vi "getDescription.vi"(8 "error in (no error)":errorcluster, 11 "Camera in":refnum<class "Camera.lvclass">) -> (0 "error out":errorcluster, 2 "description":T1={"serial"=4294967295, "type"=0, "sub_type"=0, "interface_type"=65535, "bit_resolution"=0, "min_exposure_time_s"=nan, "max_exposure_time_s"=nan, "min_exposure_step_s"=nan, "min_delay_time_s"=nan, "max_delay_time_s"=nan, "min_delay_step_s"=nan, "min_width"=18446744073709551615, "min_height"=18446744073709551615, "max_width"=18446744073709551615, "max_height"=18446744073709551615, "roi_step_horz"=18446744073709551615, "roi_step_vert"=18446744073709551615, "roi_symmetric_horz"=FALSE, "roi_symmetric_vert"=FALSE, "has_timestamp_mode"=FALSE, "has_timestamp_mode_ascii_only"=FALSE, "pixelrate_vec"=[], "conversion_factor_vec"=[], "has_trigger_mode_extexpctrl"=FALSE, "has_acquire_mode"=FALSE, "has_ext_acquire_mode"=FALSE, "has_metadata_mode"=FALSE, "has_ram"=FALSE, "binning_horz_vec"=[], "binning_vert_vec"=[], "has_average_binning"=FALSE, "pixel_format_vec"=[]} {"conversion_factor_vec" format="%.2g"; "interface_type" items=["FireWire"=1, "GenICam"=3, "GigE"=5, "USB"=6, "CameraLinkME4"=7, "USB3"=8, "CLHS"=11, "All"=65535]}, 3 "Camera out":refnum<class "Camera.lvclass">)   [LabVIEW 2019, in "Camera.lvclass"]
doc: "Gets the camera description from the camera."
uses:
  Camera.lvclass
  Camera.lvclass/Camera.ctl
  pco.sdk/CameraDescription/CameraDescription.lvlib
  pco.sdk/ImageSensor/ImageSensor.lvlib
  pco.sdk/GeneralCameraControl/GeneralCameraControl.lvlib
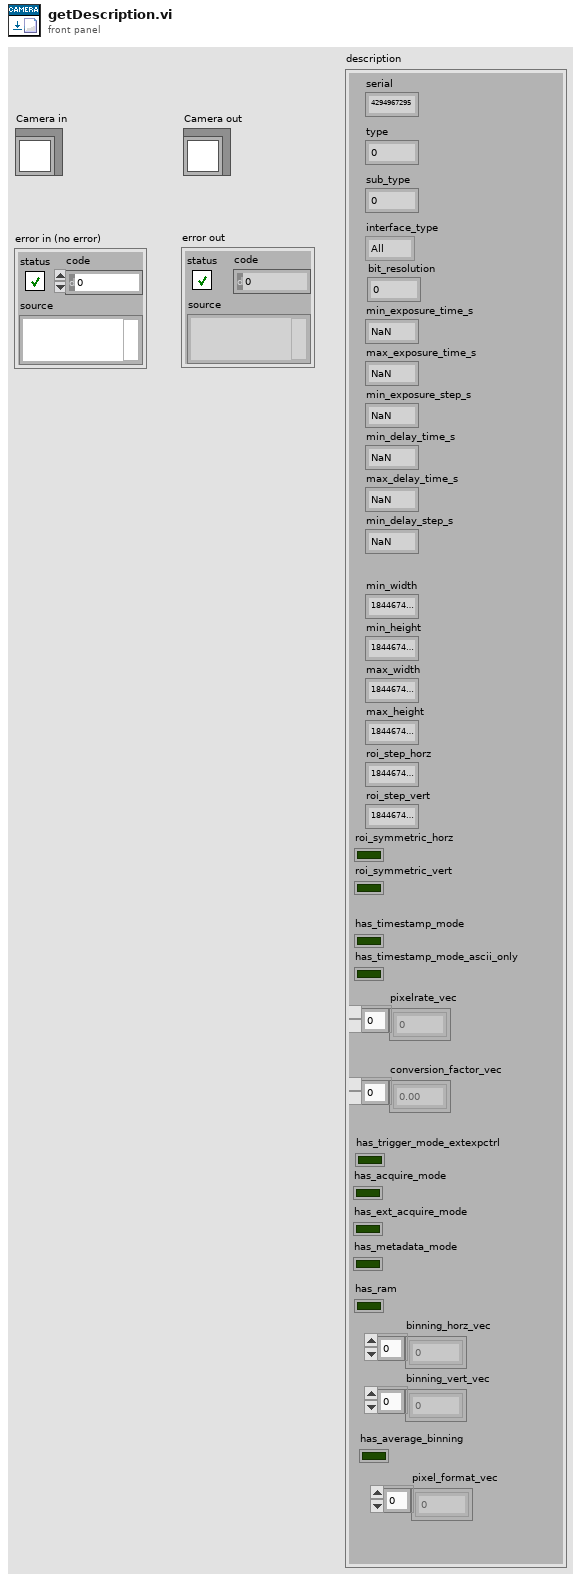
[diagram p1: front panel]
types:
  T1 = cluster{"serial":u32, "type":u16, "sub_type":u16, "interface_type":u16, "bit_resolution":u16, "min_exposure_time_s":dbl, "max_exposure_time_s":dbl, "min_exposure_step_s":dbl, "min_delay_time_s":dbl, "max_delay_time_s":dbl, "min_delay_step_s":dbl, "min_width":u64, "min_height":u64, "max_width":u64, "max_height":u64, "roi_step_horz":u64, "roi_step_vert":u64, "roi_symmetric_horz":bool, "roi_symmetric_vert":bool, "has_timestamp_mode":bool, "has_timestamp_mode_ascii_only":bool, "pixelrate_vec":u32[], "conversion_factor_vec":sgl[], "has_trigger_mode_extexpctrl":bool, "has_acquire_mode":bool, "has_ext_acquire_mode":bool, "has_metadata_mode":bool, "has_ram":bool, "binning_horz_vec":u16[], "binning_vert_vec":u16[], "has_average_binning":bool, "pixel_format_vec":u32[]}
  T2 = cluster{"serial":u32, "type":u16, "sub_type":u16, "interface_type":u16, "bit_resolution":u16, "min_exposure_time_s":dbl, "max_exposure_time_s":dbl, "min_exposure_step_s":dbl, "min_delay_time_s":dbl, "max_delay_time_s":dbl, "min_delay_step_s":dbl, "min_width":u64, "min_height":u64, "max_width":u64, "max_height":u64, "roi_step_horz":u64, "roi_step_vert":u64, "roi_symmetric_horz":bool, "roi_symmetric_vert":bool, "has_timestamp_mode":bool, "has_timestamp_mode_ascii_only":bool, "pixelrate_vec":u32[], "conversion_factor_vec":u32[], "has_trigger_mode_extexpctrl":bool, "has_acquire_mode":bool, "has_ext_acquire_mode":bool, "has_metadata_mode":bool, "has_ram":bool, "binning_horz_vec":u16[], "binning_vert_vec":u16[], "has_average_binning":bool, "pixel_format_vec":u32[]}
  T3 = enum16{"SETUP_TYPE_SHUTTERMODE", "SETUP_TYPE_PIXELFORMAT", "SETUP_TYPE_SENSOR_DYNRES"}
  T4 = cluster{"wSensorTypeDESC":u16, "wSensorSubTypeDESC":u16, "wMaxHorzResStdDESC":u16, "wMaxVertResStdDESC":u16, "wMaxHorzResExtDESC":u16, "wMaxVertResExtDESC":u16, "wDynResDESC":u16, "wMaxBinHorzDESC":u16, "wBinHorzSteppingDESC":u16, "wMaxBinVertDESC":u16, "wBinVertSteppingDESC":u16, "wRoiHorStepsDESC":u16, "wRoiVertStepsDESC":u16, "wNumADCsDESC":u16, "wMinSizeHorzDESC":u16, "dwPixelRateDESC":u32[], "wConvFactDESC":u16[], "sCoolingSetpoints":i16[], "wSoftRoiHorStepsDESC":u16, "wSoftRoiVertStepsDESC":u16, "wIRDESC":u16, "wMinSizeVertDESC":u16, "dwMinDelayDESC":u32, "dwMaxDelayDESC":u32, "dwMinDelayStepDESC":u32, "dwMinExposureDESC":u32, "dwMaxExposureDESC":u32, "dwMinExposureStepDESC":u32, "dwMinDelayIRDESC":u32, "dwMaxDelayIRDESC":u32, "dwMinExposureIRDESC":u32, "dwMaxExposureIRDESC":u32, "wTimeTableDESC":u16, "wDoubleImageDESC":u16, "sMinCoolSetDESC":i16, "sMaxCoolSetDESC":i16, "sDefaultCoolSetDESC":i16, "wPowerDownModeDESC":u16, "wOffsetRegulationDESC":u16, "wColorPatternDESC":u16, "wPatternTypeDESC":u16, "wNumCoolingSetpoints":u16, "dwGeneralCapsDESC1":u32, "dwGeneralCapsDESC2":u32, "dwExtSyncFrequency":u32[], "dwGeneralCapsDESC3":u32, "dwGeneralCapsDESC4":u32}
  T5 = cluster{"wDarkOffsetDESC3":u16, "dwGeneralCapsDESC3_1":u32, "dwGeneralCapsDESC3_2":u32, "dwGeneralCapsDESC3_3":u32, "dwGeneralCapsDESC3_4":u32, "wMinHorzResStdDESC3":u16, "wMinVertResStdDESC3":u16, "wMinHorzResExtDESC3":u16, "wMinVertResExtDESC3":u16, "dPixelsize_horzDESC3_um":dbl, "dPixelsize_vertDESC3_um":dbl, "dMinSensorTempWarningDESC3_C":dbl, "dMaxSensorTempWarningDESC3_C":dbl, "dMinCameraTempWarningDESC3_C":dbl, "dMaxCameraTempWarningDESC3_C":dbl, "dMinPowerTempWarningDESC3_C":dbl, "dMaxPowerTempWarningDESC3_C":dbl, "dMinPowerVoltageWarningDESC3_V":dbl, "dMaxPowerVoltageWarningDESC3_V":dbl, "dMinSensorTempErrorDESC3_C":dbl, "dMaxSensorTempErrorDESC3_C":dbl, "dMinCameraTempErrorDESC3_C":dbl, "dMaxCameraTempErrorDESC3_C":dbl, "dMinPowerTempErrorDESC3_C":dbl, "dMaxPowerTempErrorDESC3_C":dbl, "dMinPowerVoltageErrorDESC3_V":dbl, "dMaxPowerVoltageErrorDESC3_V":dbl}
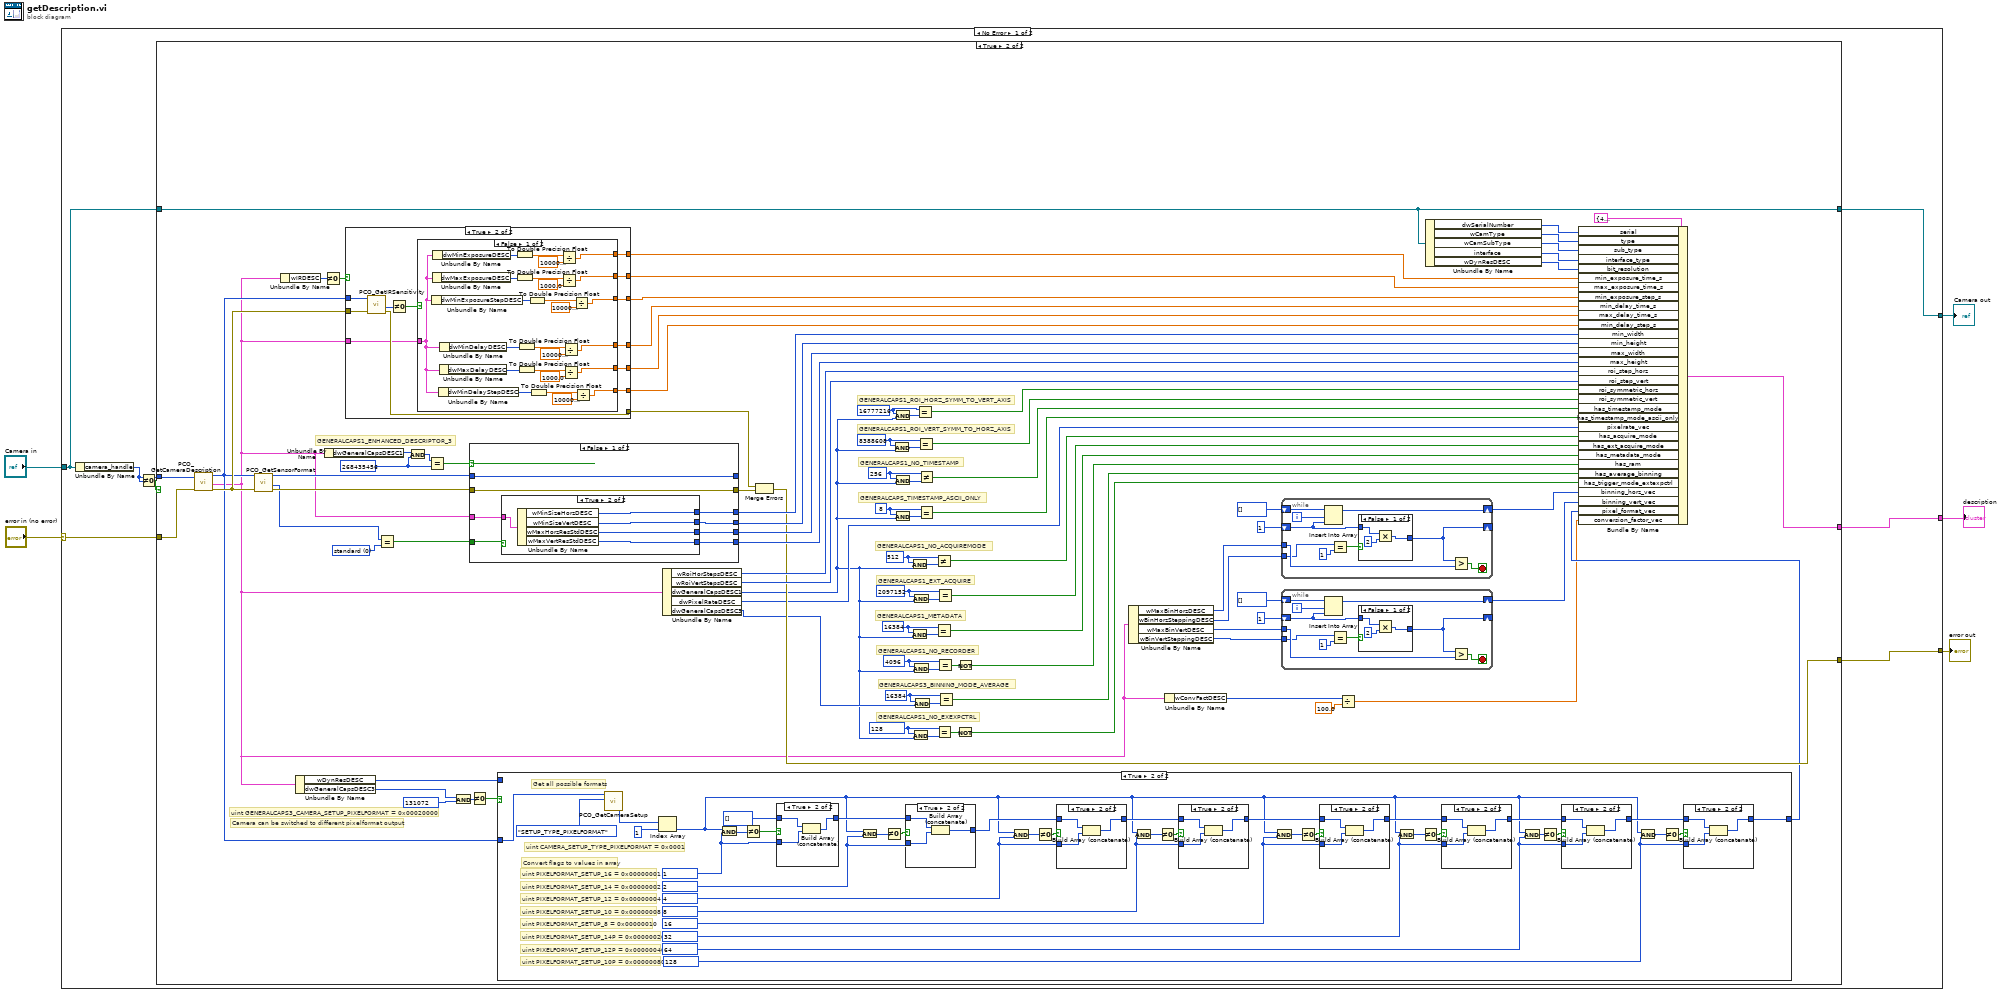
[diagram p0: block diagram]
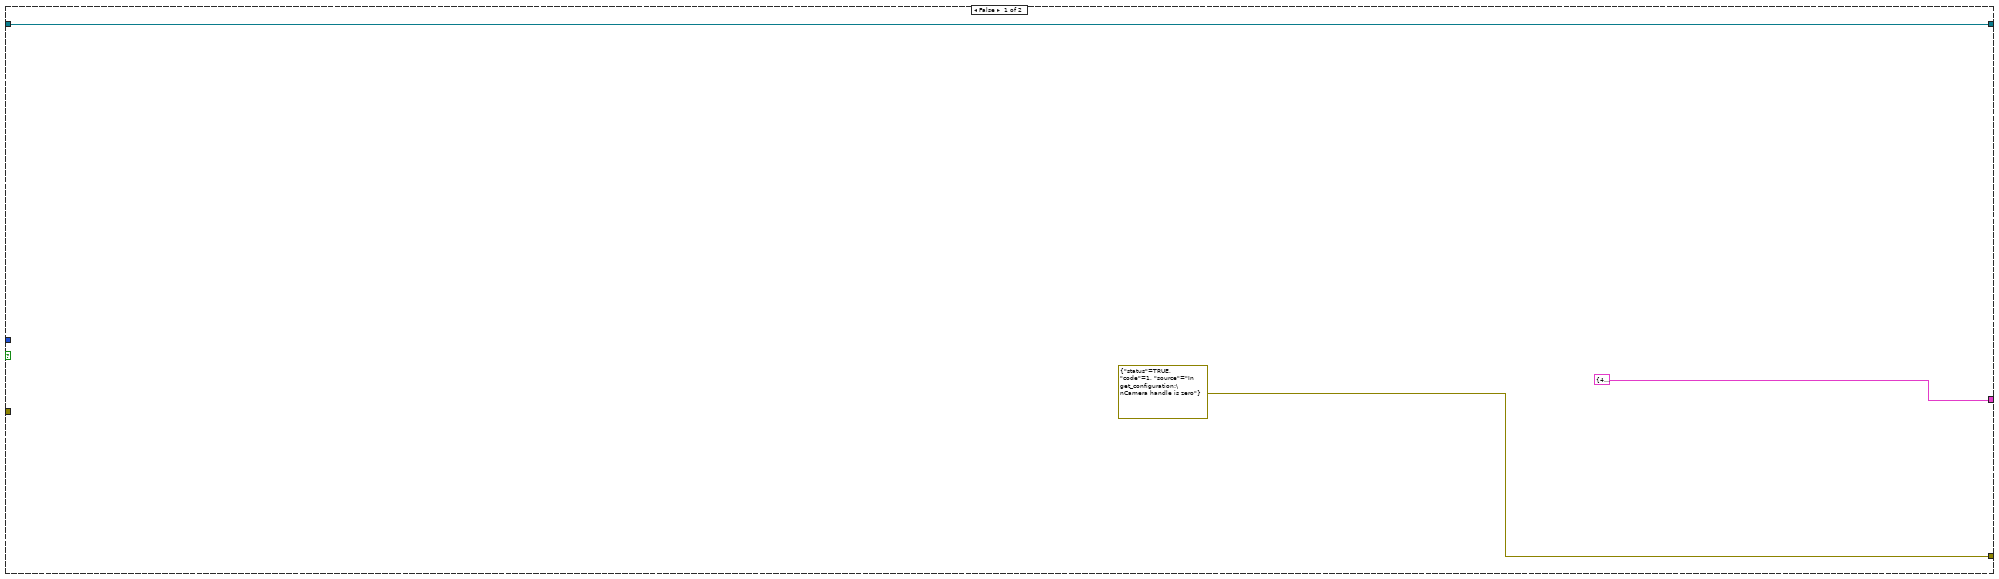
[diagram p2: hidden frame]
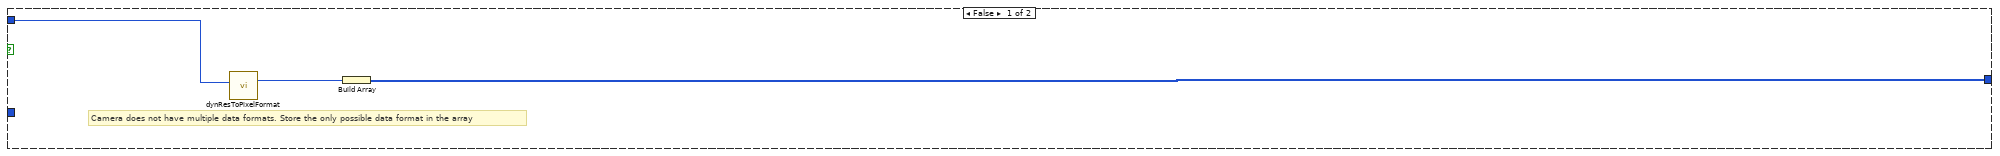
[diagram p3: hidden frame]
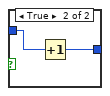
[diagram p12: hidden frame]
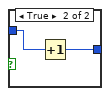
[diagram p13: hidden frame]
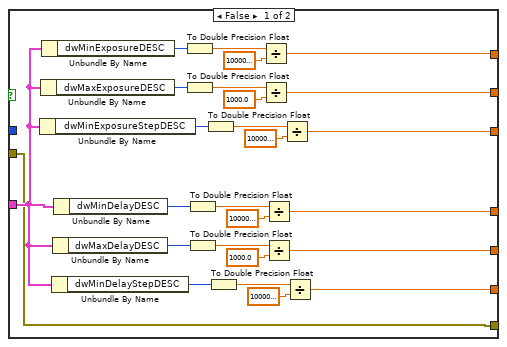
[diagram p14: hidden frame]
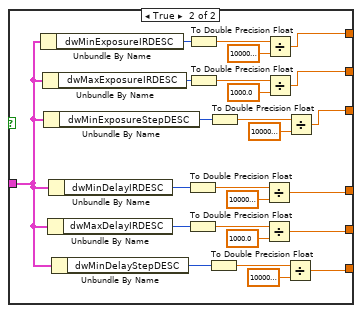
[diagram p15: hidden frame]
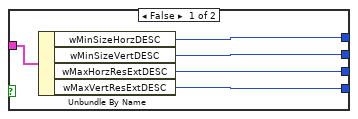
[diagram p16: hidden frame]
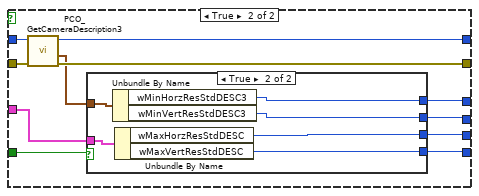
[diagram p17: hidden frame]
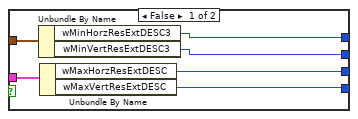
[diagram p18: hidden frame]
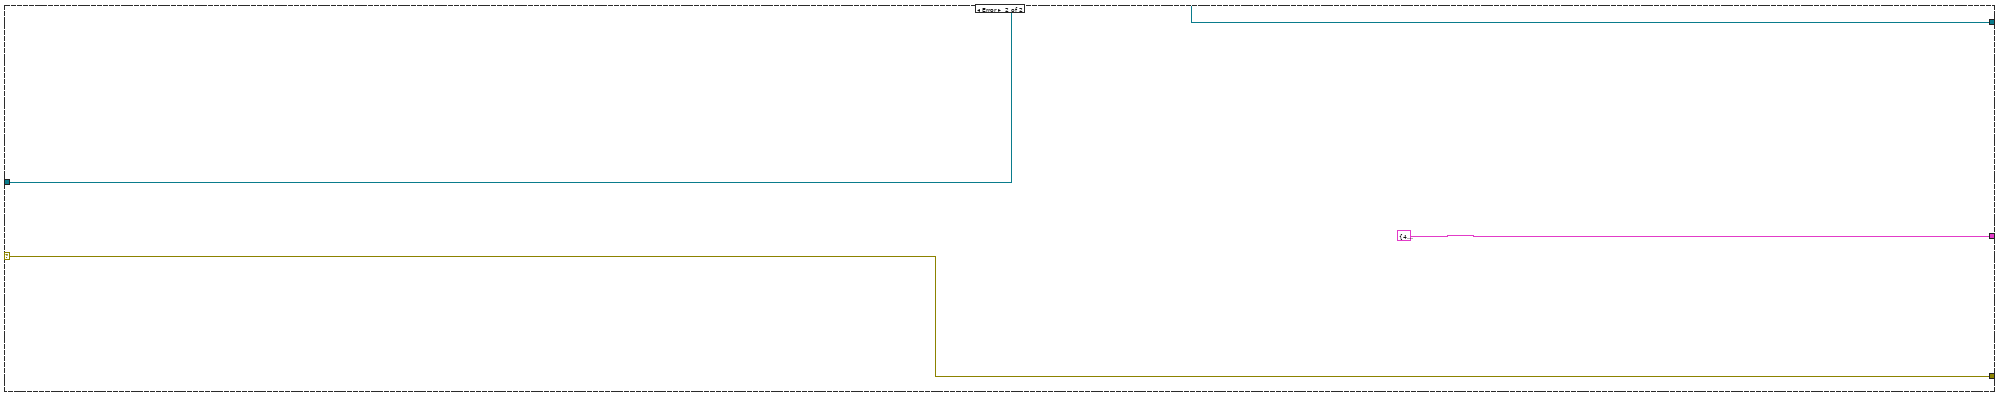
[diagram p19: hidden frame]
diagram:
  n1 = case shown="No Error" "error in (no error)" {
    selector: "error in (no error)" -> [w9 w343]
    tunnel: [w11 w343] -> w4
    tunnel: [w6 w342] -> w2
    tunnel: "Camera in" -> [w8 w342]
    tunnel: [w7 T2 {"serial"=4294967295, "type"=0, "sub_type"=0, "interface_type"=65535, "bit_resolution"=0, "min_exposure_time_s"=nan, "max_exposure_time_s"=nan, "min_exposure_step_s"=nan, "min_delay_time_s"=nan, "max_delay_time_s"=nan, "min_delay_step_s"=nan, "min_width"=18446744073709551615, "min_height"=18446744073709551615, "max_width"=18446744073709551615, "max_height"=18446744073709551615, "roi_step_horz"=18446744073709551615, "roi_step_vert"=18446744073709551615, "roi_symmetric_horz"=FALSE, "roi_symmetric_vert"=FALSE, "has_timestamp_mode"=FALSE, "has_timestamp_mode_ascii_only"=FALSE, "pixelrate_vec"=[], "conversion_factor_vec"=[], "has_trigger_mode_extexpctrl"=FALSE, "has_acquire_mode"=FALSE, "has_ext_acquire_mode"=FALSE, "has_metadata_mode"=FALSE, "has_ram"=FALSE, "binning_horz_vec"=[], "binning_vert_vec"=[], "has_average_binning"=FALSE, "pixel_format_vec"=[]} ("description")] -> w1
    frame No Error {
      n2 = Unbundle By Name(w8) -> ("camera_handle"=w10:u64)
      n3 = Not Equal To 0?(x=w10) -> (x != 0?=w12:bool)
      n4 = case shown="True" w12 {
        tunnel: [errorcluster {"status"=TRUE, "code"=1, "source"="In get_configuration:\nCamera handle is zero"} ("error constant") w68] -> w11
        tunnel: w10 -> [_ w108]
        tunnel: w9 -> [_ w107]
        tunnel: w8 -> [w14 w49]
        tunnel: [T2 {"serial"=4294967295, "type"=0, "sub_type"=0, "interface_type"=65535, "bit_resolution"=0, "min_exposure_time_s"=nan, "max_exposure_time_s"=nan, "min_exposure_step_s"=nan, "min_delay_time_s"=nan, "max_delay_time_s"=nan, "min_delay_step_s"=nan, "min_width"=18446744073709551615, "min_height"=18446744073709551615, "max_width"=18446744073709551615, "max_height"=18446744073709551615, "roi_step_horz"=18446744073709551615, "roi_step_vert"=18446744073709551615, "roi_symmetric_horz"=FALSE, "roi_symmetric_vert"=FALSE, "has_timestamp_mode"=FALSE, "has_timestamp_mode_ascii_only"=FALSE, "pixelrate_vec"=[], "conversion_factor_vec"=[], "has_trigger_mode_extexpctrl"=FALSE, "has_acquire_mode"=FALSE, "has_ext_acquire_mode"=FALSE, "has_metadata_mode"=FALSE, "has_ram"=FALSE, "binning_horz_vec"=[], "binning_vert_vec"=[], "has_average_binning"=FALSE, "pixel_format_vec"=[]} ("description") w35] -> w7
        tunnel: [w14 w49] -> w6
        frame False {
        }
        frame True {
          w24 = u32 128 ("dwGeneralCapsDESC1")
          w39 = u32 16384 ("dwGeneralCapsDESC1")
          w42 = u32 4096 ("dwGeneralCapsDESC1")
          w60 = u32 16384 ("dwGeneralCapsDESC1")
          w62 = u32 2097152 ("dwGeneralCapsDESC1")
          w66 = u32 512 ("dwGeneralCapsDESC1")
          w72 = u32 8 ("dwGeneralCapsDESC1")
          w76 = u32 256 ("dwGeneralCapsDESC1")
          w81 = u32 8388608 ("dwGeneralCapsDESC1")
          w80 = u32 16777216 ("dwGeneralCapsDESC1")
          w100 = u16 0 items=["standard", "extended"] ("wSensor")
          w104 = u32 268435456 ("dwGeneralCapsDESC1")
          # "GENERALCAPS1_NO_EXEXPCTRL"
          # "Camera can be switched to different pixelformat output"
          # "uint GENERALCAPS3_CAMERA_SETUP_PIXELFORMAT = 0x00020000"
          # "GENERALCAPS3_BINNING_MODE_AVERAGE"
          # "GENERALCAPS1_NO_RECORDER"
          # "GENERALCAPS1_METADATA"
          # "GENERALCAPS1_EXT_ACQUIRE"
          # "GENERALCAPS1_NO_ACQUIREMODE"
          # "GENERALCAPS_TIMESTAMP_ASCII_ONLY"
          # "GENERALCAPS1_NO_TIMESTAMP"
          # "GENERALCAPS1_ROI_VERT_SYMM_TO_HORZ_AXIS"
          # "GENERALCAPS1_ROI_HORZ_SYMM_TO_VERT_AXIS"
          # "GENERALCAPS1_ENHANCED_DESCRIPTOR_3"
          n5 = call "PCO_GetCameraDescription.vi"("error in (no error)"=w107, "ph"=w108) -> ("error out"=w90:errorcluster, "strDescription"=w19:T4, "ph out"=w30:u64)  [unwired: 6 in, 1 out]
          n6 = call "PCO_GetSensorFormat.vi"("error in (no error)"=w90, "ph"=w30) -> ("error out"=w102:errorcluster, "wSensor"=w99:u16, "ph out"=w101:u64)  [unwired: 6 in, 1 out]
          n7 = Unbundle By Name(w19) -> ("wIRDESC"=w98:u16)
          n8 = Unbundle By Name(w19) -> ("wDynResDESC"=w29:u16, "dwGeneralCapsDESC3"=w34:u32)
          n9 = Not Equal To 0?(x=w98) -> (x != 0?=w97:bool)
          n10 = Unbundle By Name(w19) -> ("dwGeneralCapsDESC1"=w106:u32)
          n11 = case shown="True" w97 {
            tunnel: w30 -> [_ w249]
            tunnel: w90 -> [w212 w248]
            tunnel: w19 -> [w218 w238]
            tunnel: [w234 w244] -> w96
            tunnel: [w217 w243] -> w95
            tunnel: [w216 w242] -> w94
            tunnel: [w215 w241] -> w93
            tunnel: [w214 w240] -> w92
            tunnel: [w213 w239] -> w91
            tunnel: [w212 w246] -> w70
            frame False {
              n12 = Unbundle By Name(w218) -> ("dwMinExposureStepDESC"=w228:u32)
              n13 = Unbundle By Name(w218) -> ("dwMaxExposureDESC"=w231:u32)
              n14 = Unbundle By Name(w218) -> ("dwMinExposureDESC"=w237:u32)
              n15 = Unbundle By Name(w218) -> ("dwMinDelayStepDESC"=w219:u32)
              n16 = Unbundle By Name(w218) -> ("dwMaxDelayDESC"=w222:u32)
              n17 = Unbundle By Name(w218) -> ("dwMinDelayDESC"=w227:u32)
              n18 = To Double Precision Float(number=w237) -> (double precision float=w236:dbl)
              n19 = To Double Precision Float(number=w231) -> (double precision float=w233:dbl)
              n20 = To Double Precision Float(number=w227) -> (double precision float=w226:dbl)
              n21 = To Double Precision Float(number=w222) -> (double precision float=w224:dbl)
              n22 = To Double Precision Float(number=w228) -> (double precision float=w230:dbl)
              n23 = To Double Precision Float(number=w219) -> (double precision float=w221:dbl)
              n24 = Divide(x=w236, y=1000000000.0) -> (x/y=w234:dbl)
              n25 = Divide(x=w233, y=1000.0) -> (x/y=w217:dbl)
              n26 = Divide(x=w226, y=1000000000.0) -> (x/y=w215:dbl)
              n27 = Divide(x=w224, y=1000.0) -> (x/y=w214:dbl)
              n28 = Divide(x=w230, y=1000000000.0) -> (x/y=w216:dbl)
              n29 = Divide(x=w221, y=1000000000.0) -> (x/y=w213:dbl)
            }
            frame True {
              n30 = call "PCO_GetIRSensitivity.vi"("error in (no error)"=w248, "ph"=w249) -> ("error out"=w246:errorcluster, "wIR"=w247:u16)  [unwired: 6 in, 2 out]
              n31 = Not Equal To 0?(x=w247) -> (x != 0?=w245:bool)
              n32 = case shown="False" w245 {
                tunnel: [w262 w286] -> w244
                tunnel: [w261 w285] -> w243
                tunnel: [w260 w284] -> w242
                tunnel: [w259 w283] -> w241
                tunnel: [w258 w282] -> w240
                tunnel: [w257 w281] -> w239
                tunnel: w238 -> [w250 w287]
                frame False {
                  n33 = Unbundle By Name(w250) -> ("dwMinExposureStepDESC"=w269:u32)
                  n34 = Unbundle By Name(w250) -> ("dwMaxExposureDESC"=w271:u32)
                  n35 = Unbundle By Name(w250) -> ("dwMinExposureDESC"=w274:u32)
                  n36 = Unbundle By Name(w250) -> ("dwMinDelayStepDESC"=w263:u32)
                  n37 = Unbundle By Name(w250) -> ("dwMaxDelayDESC"=w265:u32)
                  n38 = Unbundle By Name(w250) -> ("dwMinDelayDESC"=w268:u32)
                  n39 = To Double Precision Float(number=w274) -> (double precision float=w273:dbl)
                  n40 = To Double Precision Float(number=w271) -> (double precision float=w272:dbl)
                  n41 = To Double Precision Float(number=w268) -> (double precision float=w267:dbl)
                  n42 = To Double Precision Float(number=w265) -> (double precision float=w266:dbl)
                  n43 = To Double Precision Float(number=w269) -> (double precision float=w270:dbl)
                  n44 = To Double Precision Float(number=w263) -> (double precision float=w264:dbl)
                  n45 = Divide(x=w273, y=1000000000.0) -> (x/y=w262:dbl)
                  n46 = Divide(x=w272, y=1000.0) -> (x/y=w261:dbl)
                  n47 = Divide(x=w267, y=1000000000.0) -> (x/y=w259:dbl)
                  n48 = Divide(x=w266, y=1000.0) -> (x/y=w258:dbl)
                  n49 = Divide(x=w270, y=1000000000.0) -> (x/y=w260:dbl)
                  n50 = Divide(x=w264, y=1000000000.0) -> (x/y=w257:dbl)
                }
                frame True {
                  n51 = Unbundle By Name(w287) -> ("dwMinExposureIRDESC"=w299:u32)
                  n52 = Unbundle By Name(w287) -> ("dwMaxExposureIRDESC"=w296:u32)
                  n53 = Unbundle By Name(w287) -> ("dwMinExposureStepDESC"=w294:u32)
                  n54 = Unbundle By Name(w287) -> ("dwMaxDelayIRDESC"=w290:u32)
                  n55 = Unbundle By Name(w287) -> ("dwMinDelayIRDESC"=w293:u32)
                  n56 = Unbundle By Name(w287) -> ("dwMinDelayStepDESC"=w288:u32)
                  n57 = To Double Precision Float(number=w293) -> (double precision float=w292:dbl)
                  n58 = To Double Precision Float(number=w290) -> (double precision float=w291:dbl)
                  n59 = To Double Precision Float(number=w299) -> (double precision float=w298:dbl)
                  n60 = To Double Precision Float(number=w296) -> (double precision float=w297:dbl)
                  n61 = To Double Precision Float(number=w288) -> (double precision float=w289:dbl)
                  n62 = To Double Precision Float(number=w294) -> (double precision float=w295:dbl)
                  n63 = Divide(x=w292, y=1000000000.0) -> (x/y=w283:dbl)
                  n64 = Divide(x=w291, y=1000.0) -> (x/y=w282:dbl)
                  n65 = Divide(x=w298, y=1000000000.0) -> (x/y=w286:dbl)
                  n66 = Divide(x=w297, y=1000.0) -> (x/y=w285:dbl)
                  n67 = Divide(x=w289, y=1000000000.0) -> (x/y=w281:dbl)
                  n68 = Divide(x=w295, y=1000000000.0) -> (x/y=w284:dbl)
                }
              }
            }
          }
          n69 = Equal?(x=w99, y=w100) -> (x = y?=w89:bool)
          n70 = And(x=w106, y=w104) -> (x .and. y?=w105:u32)
          n71 = Equal?(x=w105, y=w104) -> (x = y?=w103:bool)
          n72 = And(x=w34, y=u32 131072) -> (x .and. y?=w32:u32)
          n73 = case shown="False" w103 {
            tunnel: w102 -> [w307 w328]
            tunnel: w101 -> [w306 w327]
            tunnel: w19 -> [w304 w323]
            tunnel: [w307 w325] -> w69
            tunnel: [w306 w326] -> _
            tunnel: w89 -> [w305 w324]
            tunnel: [w303 w321] -> w88
            tunnel: [w302 w320] -> w87
            tunnel: [w301 w319] -> w86
            tunnel: [w300 w318] -> w85
            frame False {
              n74 = case shown="True" w305 {
                tunnel: w304 -> [w312 w317]
                tunnel: [w308 w316] -> w303
                tunnel: [w309 w315] -> w302
                tunnel: [w310 w314] -> w301
                tunnel: [w311 w313] -> w300
                frame False {
                  n75 = Unbundle By Name(w312) -> ("wMinSizeHorzDESC"=w308:u16, "wMinSizeVertDESC"=w309:u16, "wMaxHorzResExtDESC"=w310:u16, "wMaxVertResExtDESC"=w311:u16)
                }
                frame True {
                  n76 = Unbundle By Name(w317) -> ("wMinSizeHorzDESC"=w316:u16, "wMinSizeVertDESC"=w315:u16, "wMaxHorzResStdDESC"=w314:u16, "wMaxVertResStdDESC"=w313:u16)
                }
              }
            }
            frame True {
              n77 = call "PCO_GetCameraDescription3.vi"("error in (no error)"=w328, "ph"=w327) -> ("error out"=w325:errorcluster, "strDescription"=w322:T5, "ph out"=w326:u64)  [unwired: 6 in, 1 out]
              n78 = case shown="True" w324 {
                tunnel: w323 -> [w333 w340]
                tunnel: [w329 w336] -> w321
                tunnel: [w330 w335] -> w320
                tunnel: [w331 w339] -> w319
                tunnel: [w332 w338] -> w318
                tunnel: w322 -> [w334 w337]
                frame False {
                  n79 = Unbundle By Name(w334) -> ("wMinHorzResExtDESC3"=w329:u16, "wMinVertResExtDESC3"=w330:u16)
                  n80 = Unbundle By Name(w333) -> ("wMaxHorzResExtDESC"=w331:u16, "wMaxVertResExtDESC"=w332:u16)
                }
                frame True {
                  n81 = Unbundle By Name(w337) -> ("wMinHorzResStdDESC3"=w336:u16, "wMinVertResStdDESC3"=w335:u16)
                  n82 = Unbundle By Name(w340) -> ("wMaxHorzResStdDESC"=w339:u16, "wMaxVertResStdDESC"=w338:u16)
                }
              }
            }
          }
          n83 = Not Equal To 0?(x=w32) -> (x != 0?=w31:bool)
          n84 = case shown="True" w31 {
            tunnel: w30 -> [_ w147]
            tunnel: [w109 w113] -> w28
            tunnel: w29 -> [w111 _]
            frame False {
              # "Camera does not have multiple data formats. Store the only possible data format in the array"
              n85 = call "dynResToPixelFormat.vi"("dyn_res"=w111) -> ("PixelFormat"=w110:u32)  [unwired: 9 in, 1 out]
              n86 = Build Array(w110) -> (w109:u32[])
            }
            frame True {
              w114 = u32 128
              w115 = u32 64
              w123 = u32 32
              w124 = u32 16
              w131 = u32 8
              w135 = u32 4
              w140 = u32 2
              w143 = u32 1
              # "Convert flags to values in array"
              # "Get all possible formats"
              # "uint PIXELFORMAT_SETUP_10P = 0x00000080"
              # "uint PIXELFORMAT_SETUP_12P = 0x00000040"
              # "uint PIXELFORMAT_SETUP_14P = 0x00000020"
              # "uint PIXELFORMAT_SETUP_8 = 0x00000010"
              # "uint PIXELFORMAT_SETUP_10 = 0x00000008"
              # "uint PIXELFORMAT_SETUP_12 = 0x00000004"
              # "uint PIXELFORMAT_SETUP_14 = 0x00000002"
              # "uint PIXELFORMAT_SETUP_16 = 0x00000001"
              # "uint CAMERA_SETUP_TYPE_PIXELFORMAT = 0x0001"
              n87 = call "PCO_GetCameraSetup.vi"("wTypeIn"=T3."SETUP_TYPE_PIXELFORMAT", "ph"=w147) -> ("dwSetup"=w149:u32[])  [unwired: 5 in, 4 out]
              n88 = Index Array(array=w149, index=1) -> (element=w116:u32)
              n89 = And(x=w116, y=w143) -> (x .and. y?=w146:u32)
              n90 = Not Equal To 0?(x=w146) -> (x != 0?=w145:bool)
              n91 = case shown="True" w145 {
                tunnel: u32[] [] -> [w178 w181]
                tunnel: w143 -> [_ w180]
                tunnel: [w178 w179] -> w139
                frame False {
                }
                frame True {
                  n92 = Build Array (concatenate)(w181, w180) -> (w179:u32[])
                }
              }
              n93 = And(x=w116, y=w140) -> (x .and. y?=w142:u32)
              n94 = Not Equal To 0?(x=w142) -> (x != 0?=w141:bool)
              n95 = case shown="True" w141 {
                tunnel: w139 -> [w174 w177]
                tunnel: w140 -> [_ w176]
                tunnel: [w174 w175] -> w136
                frame False {
                }
                frame True {
                  n96 = Build Array (concatenate)(w177, w176) -> (w175:u32[])
                }
              }
              n97 = And(x=w116, y=w135) -> (x .and. y?=w137:u32)
              n98 = Not Equal To 0?(x=w137) -> (x != 0?=w138:bool)
              n99 = case shown="True" w138 {
                tunnel: w136 -> [w170 w173]
                tunnel: w135 -> [_ w172]
                tunnel: [w170 w171] -> w132
                frame False {
                }
                frame True {
                  n100 = Build Array (concatenate)(w173, w172) -> (w171:u32[])
                }
              }
              n101 = And(x=w116, y=w131) -> (x .and. y?=w134:u32)
              n102 = Not Equal To 0?(x=w134) -> (x != 0?=w133:bool)
              n103 = case shown="True" w133 {
                tunnel: w132 -> [w166 w169]
                tunnel: w131 -> [_ w168]
                tunnel: [w166 w167] -> w125
                frame False {
                }
                frame True {
                  n104 = Build Array (concatenate)(w169, w168) -> (w167:u32[])
                }
              }
              n105 = And(x=w116, y=w124) -> (x .and. y?=w127:u32)
              n106 = Not Equal To 0?(x=w127) -> (x != 0?=w126:bool)
              n107 = case shown="True" w126 {
                tunnel: w125 -> [w162 w165]
                tunnel: w124 -> [_ w164]
                tunnel: [w162 w163] -> w130
                frame False {
                }
                frame True {
                  n108 = Build Array (concatenate)(w165, w164) -> (w163:u32[])
                }
              }
              n109 = And(x=w116, y=w123) -> (x .and. y?=w128:u32)
              n110 = Not Equal To 0?(x=w128) -> (x != 0?=w129:bool)
              n111 = case shown="True" w129 {
                tunnel: w130 -> [w158 w161]
                tunnel: w123 -> [_ w160]
                tunnel: [w158 w159] -> w117
                frame False {
                }
                frame True {
                  n112 = Build Array (concatenate)(w161, w160) -> (w159:u32[])
                }
              }
              n113 = And(x=w116, y=w115) -> (x .and. y?=w121:u32)
              n114 = Not Equal To 0?(x=w121) -> (x != 0?=w122:bool)
              n115 = case shown="True" w122 {
                tunnel: w117 -> [w154 w157]
                tunnel: w115 -> [_ w156]
                tunnel: [w154 w155] -> w118
                frame False {
                }
                frame True {
                  n116 = Build Array (concatenate)(w157, w156) -> (w155:u32[])
                }
              }
              n117 = And(x=w116, y=w114) -> (x .and. y?=w120:u32)
              n118 = Not Equal To 0?(x=w120) -> (x != 0?=w119:bool)
              n119 = case shown="True" w119 {
                tunnel: w118 -> [w150 w153]
                tunnel: w114 -> [_ w152]
                tunnel: [w150 w151] -> w113
                frame False {
                }
                frame True {
                  n120 = Build Array (concatenate)(w153, w152) -> (w151:u32[])
                }
              }
            }
          }
          n121 = Unbundle By Name(w19) -> ("wRoiHorStepsDESC"=w84:u16, "wRoiVertStepsDESC"=w83:u16, "dwGeneralCapsDESC1"=w22:u32, "dwPixelRateDESC"=w67:u32[], "dwGeneralCapsDESC3"=w37:u32)
          n122 = Merge Errors(w70, w69) -> (w68:errorcluster)
          n123 = And(x=w81, y=w22) -> (x .and. y?=w82:u32)
          n124 = And(x=w80, y=w22) -> (x .and. y?=w79:u32)
          n125 = And(x=w76, y=w22) -> (x .and. y?=w75:u32)
          n126 = And(x=w72, y=w22) -> (x .and. y?=w73:u32)
          n127 = And(x=w66, y=w22) -> (x .and. y?=w65:u32)
          n128 = And(x=w60, y=w22) -> (x .and. y?=w59:u32)
          n129 = And(x=w24, y=w22) -> (x .and. y?=w23:u32)
          n130 = And(x=w62, y=w22) -> (x .and. y?=w63:u32)
          n131 = And(x=w42, y=w22) -> (x .and. y?=w43:u32)
          n132 = And(x=w39, y=w37) -> (x .and. y?=w38:u32)
          n133 = Equal?(x=w80, y=w79) -> (x = y?=w78:bool)
          n134 = Equal?(x=w81, y=w82) -> (x = y?=w77:bool)
          n135 = Not Equal?(x=w76, y=w75) -> (x != y?=w74:bool)
          n136 = Equal?(x=w72, y=w73) -> (x = y?=w71:bool)
          n137 = Not Equal?(x=w66, y=w65) -> (x != y?=w64:bool)
          n138 = Equal?(x=w60, y=w59) -> (x = y?=w58:bool)
          n139 = Equal?(x=w24, y=w23) -> (x = y?=w25:bool)
          n140 = Equal?(x=w62, y=w63) -> (x = y?=w61:bool)
          n141 = Equal?(x=w42, y=w43) -> (x = y?=w41:bool)
          n142 = Equal?(x=w39, y=w38) -> (x = y?=w36:bool)
          n143 = Not(x=w25) -> (.not. x?=w21:bool)
          n144 = Not(x=w41) -> (.not. x?=w40:bool)
          n145 = Unbundle By Name(w19) -> ("wMaxBinHorzDESC"=w57:u16, "wBinHorzSteppingDESC"=w56:u16, "wMaxBinVertDESC"=w51:u16, "wBinVertSteppingDESC"=w50:u16)
          n146 = Unbundle By Name(w19) -> ("wConvFactDESC"=w18:u16[])
          n147 = while {
            tunnel: w57 -> [w202]
            tunnel: w56 -> [w201]
            shift-right: [w204] -> w26
            shift-left: u16[] [] ("binning_horz_vec") -> [w206]
            shift-right: [w197] -> _
            shift-left: u16 1 -> [w198]
            i -> [w205]
            stop <- w203 stop-if-true
            n148 = Insert Into Array(array=w206, index=w205, new element=w198) -> (w204:u16[])
            n149 = Equal?(x=w201, y=u16 1 ("wBinHorzSteppingDESC")) -> (x = y?=w199:bool)
            n150 = case shown="False" w199 {
              tunnel: w198 -> [w208 w211]
              tunnel: [w209 w210] -> w197
              frame False {
                n151 = Multiply(x=w208, y=u16 2) -> (x*y=w209:u16)
              }
              frame True {
                n152 = Increment(x=w211) -> (x+1=w210:u16)
              }
            }
            n153 = Greater?(x=w197, y=w202) -> (0:w203:bool)
          }
          n154 = while {
            tunnel: w51 -> [w187]
            tunnel: w50 -> [w186]
            shift-right: [w189] -> w27
            shift-left: u16[] [] ("binning_horz_vec") -> [w191]
            shift-right: [w182] -> _
            shift-left: u16 1 -> [w183]
            i -> [w190]
            stop <- w188 stop-if-true
            n155 = Insert Into Array(array=w191, index=w190, new element=w183) -> (w189:u16[])
            n156 = Equal?(x=w186, y=u16 1 ("wBinHorzSteppingDESC")) -> (x = y?=w184:bool)
            n157 = case shown="False" w184 {
              tunnel: w183 -> [w193 w196]
              tunnel: [w194 w195] -> w182
              frame False {
                n158 = Multiply(x=w193, y=u16 2) -> (x*y=w194:u16)
              }
              frame True {
                n159 = Increment(x=w196) -> (x+1=w195:u16)
              }
            }
            n160 = Greater?(x=w182, y=w187) -> (0:w188:bool)
          }
          n161 = Divide(x=w18, y=sgl 100.0) -> (x/y=w17:sgl[])
          n162 = Unbundle By Name(w49) -> ("dwSerialNumber"=w48:u32, "wCamType"=w47:u16, "wCamSubType"=w46:u16, "interface"=w45:u16, "wDynResDESC"=w44:u16)
          n163 = Bundle By Name(cluster=T1 {"serial"=4294967295, "type"=0, "sub_type"=0, "interface_type"=65535, "bit_resolution"=0, "min_exposure_time_s"=nan, "max_exposure_time_s"=nan, "min_exposure_step_s"=nan, "min_delay_time_s"=nan, "max_delay_time_s"=nan, "min_delay_step_s"=nan, "min_width"=18446744073709551615, "min_height"=18446744073709551615, "max_width"=18446744073709551615, "max_height"=18446744073709551615, "roi_step_horz"=18446744073709551615, "roi_step_vert"=18446744073709551615, "roi_symmetric_horz"=FALSE, "roi_symmetric_vert"=FALSE, "has_timestamp_mode"=FALSE, "has_timestamp_mode_ascii_only"=FALSE, "pixelrate_vec"=[], "conversion_factor_vec"=[], "has_trigger_mode_extexpctrl"=FALSE, "has_acquire_mode"=FALSE, "has_ext_acquire_mode"=FALSE, "has_metadata_mode"=FALSE, "has_ram"=FALSE, "binning_horz_vec"=[], "binning_vert_vec"=[], "has_average_binning"=FALSE, "pixel_format_vec"=[]} ("description"), "serial"=w48, "type"=w47, "sub_type"=w46, "interface_type"=w45, "bit_resolution"=w44, "min_exposure_time_s"=w96, "max_exposure_time_s"=w95, "min_exposure_step_s"=w94, "min_delay_time_s"=w93, "max_delay_time_s"=w92, "min_delay_step_s"=w91, "min_width"=w88, "min_height"=w87, "max_width"=w86, "max_height"=w85, "roi_step_horz"=w84, "roi_step_vert"=w83, "roi_symmetric_horz"=w78, "roi_symmetric_vert"=w77, "has_timestamp_mode"=w74, "has_timestamp_mode_ascii_only"=w71, "pixelrate_vec"=w67, "has_acquire_mode"=w64, "has_ext_acquire_mode"=w61, "has_metadata_mode"=w58, "has_ram"=w40, "has_average_binning"=w36, "has_trigger_mode_extexpctrl"=w21, "binning_horz_vec"=w26, "binning_vert_vec"=w27, "pixel_format_vec"=w28, "conversion_factor_vec"=w17) -> (w35:T1)
        }
      }
    }
    frame Error {
    }
  }
  "error out" <- w4
  "Camera out" <- w2
  "description" <- w1
